vi "WT1800 Convert Measurement Data.vi"(8 "error in (no error)":errorcluster, 9 "Item Number Offset (1)":i32=1 min=1 max=255, 10 "Measurement Data (Empty)":string, 11 "VISA resource name":refnum<visa-resource-name>) -> (0 "error out":errorcluster, 1 "Measurement":dbl[](array[numeric]), 2 "Function":string[](array[string]), 3 "VISA resource name out":refnum<visa-resource-name>)   [LabVIEW 2021]
uses:
  <instrlib>/Yokogawa WT1800 Series/Public/Action-Status/Query Numeric (Normal).vi
  <instrlib>/Yokogawa WT1800 Series/Yokogawa WT1800 Series.lvlib
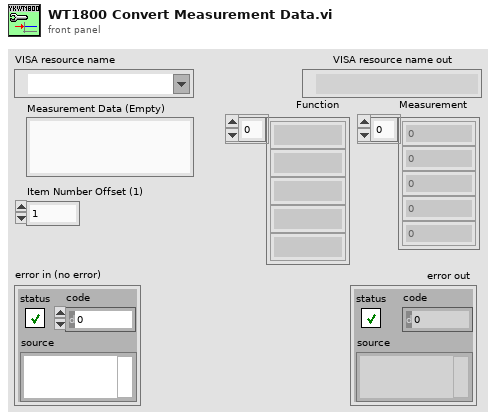
[diagram p1: front panel]
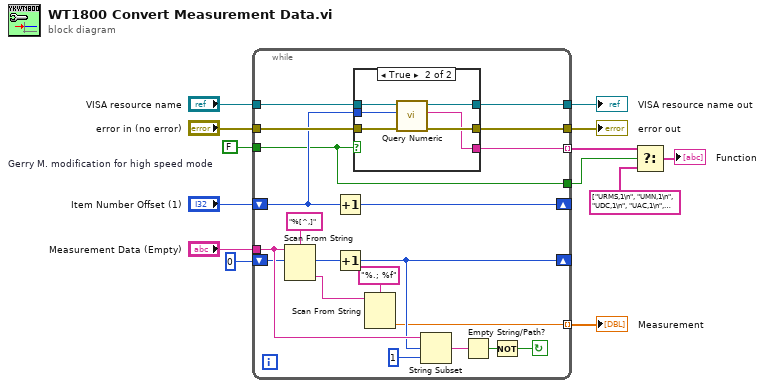
[diagram p0: block diagram]
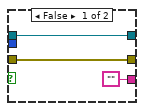
[diagram p2: hidden frame]
diagram:
  w13 = FALSE  # Gerry M. modification for high speed mode
  n1 = while {
    tunnel: [w23] -> w7 mode=indexing
    tunnel: "Measurement Data (Empty)" -> [w28]
    shift-right: [w25] -> _
    shift-left: 0 -> [w27]
    tunnel: "VISA resource name" -> [w21]
    tunnel: "error in (no error)" -> [w20]
    shift-right: [w18] -> _
    shift-left: "Item Number Offset (1)" -> [w19]
    tunnel: [w17] -> w5
    tunnel: [w16] -> w6
    tunnel: [w15] -> w10 mode=indexing
    tunnel: [w14] -> w12
    tunnel: w13 -> [w14]
    stop <- w30 continue-if-true
    n2 = Scan From String(format string="%[^,]", input string=w28, initial scan location=w27) -> (offset past scan=w26:u32, output 1=w24:string)  [unwired: 2 in, 2 out]
    n3 = Increment(x=w19) -> (x+1=w18:i32)
    n4 = Increment(x=w26) -> (x+1=w25:u32)
    n5 = case shown="True" w14 {
      tunnel: w21 -> [w36 w42]
      tunnel: w20 -> [w35 w41]
      tunnel: w19 -> [_ w40]
      tunnel: [w36 w39] -> w17
      tunnel: [w35 w38] -> w16
      tunnel: ["" ("Function") w37] -> w15
      frame False {
      }
      frame True {
        n6 = call-poly <instrlib>:"Query Numeric.vi"("error in (no error)"=w41, "Item (1)"=w40, "VISA resource name"=w42) -> ("error out"=w38:errorcluster, "Function"=w37:string, "VISA resource name out"=w39:refnum<visa-resource-name>)  [unwired: 6 in]
      }
    }
    n7 = Scan From String(format string="%.; %f" ("形式文字列"), input string=w24) -> (output 1=w23:dbl)  [unwired: 3 in, 3 out]
    n8 = String Subset(string=w28, offset (0)=w25, length (rest)=1) -> (substring=w32:string)
    n9 = Empty String/Path?(string/path=w32) -> (empty?=w31:bool)
    n10 = Not(x=w31) -> (.not. x?=w30:bool)
  }
  "error out" <- w6
  "VISA resource name out" <- w5
  "Measurement" <- w7
  n11 = Select(t=w10, s=w12, f=string[] ["URMS,1\n", "UMN,1\n", "UDC,1\n", "UAC,1\n", "IRMS,1\n", "IMN,1\n", "IDC,1\n", "IAC,1\n", "P,1\n", "S,1\n", "Q,1\n", "LAMB,1\n", "PHI,1\n", "FU,1\n", "FI,1\n", "UPP,1\n", "UMP,1\n", "IPP,1\n", "IMP,1\n", "NONE\n", "URMS,2\n", "UMN,2\n", "UDC,2\n", "UAC,2\n", "IRMS,2\n", "IMN,2\n", "IDC,2\n", "IAC,2\n", "P,2\n", "S,2\n", "Q,2\n", "LAMB,2\n", "PHI,2\n", "FU,2\n", "FI,2\n", "UPP,2\n", "UMP,2\n", "IPP,2\n", "IMP,2\n", "NONE\n", "URMS,3\n", "UMN,3\n", "UDC,3\n", "UAC,3\n", "IRMS,3\n", "IMN,3\n", "IDC,3\n", "IAC,3\n", "P,3\n", "S,3\n", "Q,3\n", "LAMB,3\n", "PHI,3\n", "FU,3\n", "FI,3\n", "UPP,3\n", "UMP,3\n", "IPP,3\n", "IMP,3\n", "NONE\n", "URMS,4\n", "UMN,4\n", "UDC,4\n", "UAC,4\n", "IRMS,4\n", "IMN,4\n", "IDC,4\n", "IAC,4\n", "P,4\n", "S,4\n", "Q,4\n", "LAMB,4\n", "PHI,4\n", "FU,4\n", "FI,4\n", "UPP,4\n", "UMP,4\n", "IPP,4\n", "IMP,4\n", "NONE\n", "URMS,5\n", "UMN,5\n", "UDC,5\n", "UAC,5\n", "IRMS,5\n", "IMN,5\n", "IDC,5\n", "IAC,5\n", "P,5\n", "S,5\n", "Q,5\n", "LAMB,5\n", "PHI,5\n", "FU,5\n", "FI,5\n", "UPP,5\n", "UMP,5\n", "IPP,5\n", "IMP,5\n", "NONE\n", "URMS,6\n", "UMN,6\n", "UDC,6\n", "UAC,6\n", "IRMS,6\n", "IMN,6\n", "IDC,6\n", "IAC,6\n", "P,6\n", "S,6\n", "Q,6\n", "LAMB,6\n", "PHI,6\n", "FU,6\n", "FI,6\n", "UPP,6\n", "UMP,6\n", "IPP,6\n", "IMP,6\n"] ("Function")) -> (s? t:f=→"Function":string[])
